vi "rvc Rotation Matrix to RPY.vi"(9 "type of rotations":u16(ring) items=["Extrinsic", "Intrinsic"], 10 "Convension":u16(ring) items=["XYZ", "ZYX"], 11 "rotation matrix":T1) -> (3 "angles":cluster{"roll":dbl, "pitch":dbl, "yaw":dbl})   [LabVIEW 2013]
uses:
  <vilib>/Analysis/Matrix/Datatypes/RealMatrix.ctl
  <vilib>/Analysis/coordinate.llb/Euler Rotation Order.ctl
  <vilib>/robotics/Kinematics/NI_Kinematics.lvlib
  <vilib>/Analysis/NI_AALBase.lvlib
  <vilib>/Analysis/baseanly.llb/Real A x B.vi
  <vilib>/Analysis/NI_AALPro.lvlib
  <vilib>/Analysis/Matrix/NI_Matrix.lvlib
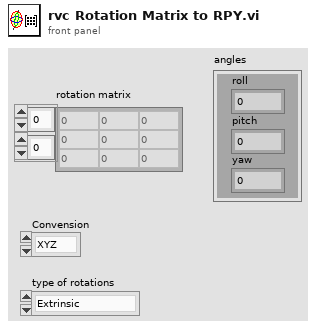
[diagram p1: front panel]
types:
  T1 = typedef "NI_Matrix.lvlib/RealMatrix.ctl" = dbl[][]
  T2 = typedef "NI_AALPro.lvlib/Euler Rotation Order.ctl" = u16
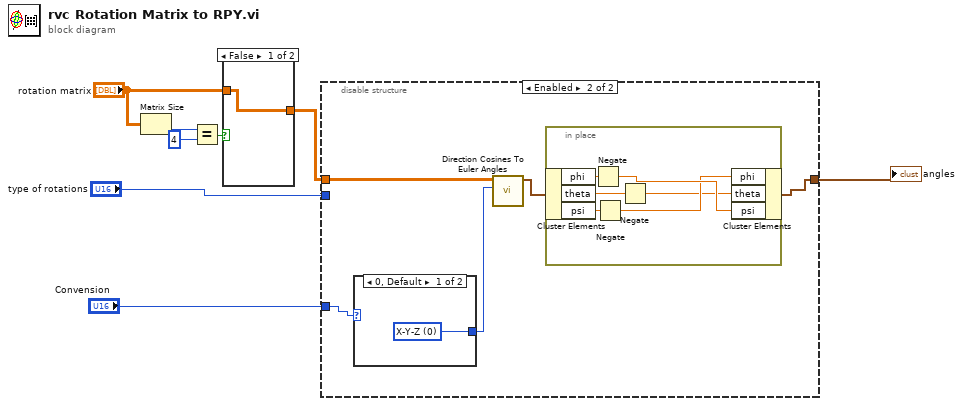
[diagram p0: block diagram]
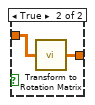
[diagram p2: hidden frame]
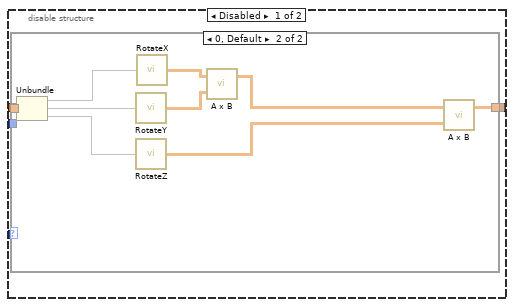
[diagram p3: hidden frame]
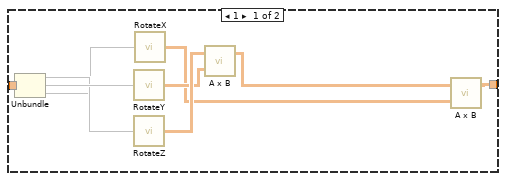
[diagram p4: hidden frame]
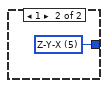
[diagram p5: hidden frame]
diagram:
  n1 = Matrix Size(0:"rotation matrix") -> (2:w5:i32)  [unwired: 1 out]
  n2 = Equal?(x=w5, y=4) -> (x = y?=w3:bool)
  n3 = case shown="False" w3 {
    tunnel: "rotation matrix" -> [w9 w11]
    tunnel: [w9 w10] -> w1
    frame False {
    }
    frame True {
      n4 = call <vilib>:"Transform to Rotation Matrix.vi"("transform"=w11) -> ("rotation matrix"=w10:T1)
    }
  }
  n5 = disable-structure shown="Enabled" {
    disable-tunnel: w1 -> [w14 w36]
    disable-tunnel: [w13 w33] -> w6
    disable-tunnel: "Convension" -> [w12 w37]
    disable-tunnel: "type of rotations" -> [_ _]
    frame Disabled {
      n6 = case shown="0, Default" w12 {
        tunnel: w14 -> [w23 w32]
        tunnel: [w21 w26] -> w13
        frame 1 {
          n7 = Unbundle(w23) -> (w16, w22, w15)
          n8 = call <vilib>:"RotateY.vi"("theta"=w22) -> ("rotation matrix"=w19:T1)
          n9 = call <vilib>:"RotateZ.vi"("theta"=w16) -> ("rotation matrix"=w20:T1)
          n10 = call <vilib>:"RotateX.vi"("theta"=w15) -> ("rotation matrix"=w17:T1)
          n11 = call-poly <vilib>:"A x B.vi"("B"=w19, "A"=w20) -> ("A x B"=w18:T1)  [unwired: 1 out]
          n12 = call-poly <vilib>:"A x B.vi"("B"=w17, "A"=w18) -> ("A x B"=w21:T1)  [unwired: 1 out]
        }
        frame 0, Default {
          n13 = Unbundle(w32) -> (w25, w31, w24)
          n14 = call <vilib>:"RotateY.vi"("theta"=w31) -> ("rotation matrix"=w29:T1)
          n15 = call <vilib>:"RotateZ.vi"("theta"=w24) -> ("rotation matrix"=w28:T1)
          n16 = call <vilib>:"RotateX.vi"("theta"=w25) -> ("rotation matrix"=w30:T1)
          n17 = call-poly <vilib>:"A x B.vi"("B"=w29, "A"=w30) -> ("A x B"=w27:T1)  [unwired: 1 out]
          n18 = call-poly <vilib>:"A x B.vi"("B"=w28, "A"=w27) -> ("A x B"=w26:T1)  [unwired: 1 out]
        }
      }
    }
    frame Enabled {
      n19 = case shown="0, Default" w37 {
        tunnel: [w44 w45] -> w35
        frame 0, Default {
          w44 = T2 0 items=["X-Y-Z", "X-Z-Y", "Y-X-Z", "Y-Z-X", "Z-X-Y", "Z-Y-X", "X-Y-X", "X-Z-X", "Y-X-Y", "Y-Z-Y", "Z-X-Z", "Z-Y-Z"] ("rotation order")
        }
        frame 1 {
          w45 = T2 5 items=["X-Y-Z", "X-Z-Y", "Y-X-Z", "Y-Z-X", "Z-X-Y", "Z-Y-X", "X-Y-X", "X-Z-X", "Y-X-Y", "Y-Z-Y", "Z-X-Z", "Z-Y-Z"] ("rotation order")
        }
      }
      n20 = call <vilib>:"Direction Cosines To Euler Angles.vi"("rotation order"=w35, "Direction Cosines"=w36) -> ("Euler Angles"=w34:cluster{"phi":dbl, "theta":dbl, "psi":dbl})  [unwired: 8 in, 1 out]
      n21 = in-place {
        n22 = in-place-cluster #1(w34) -> ("phi"=w43:dbl, "theta"=w39:dbl, "psi"=w42:dbl)
        n23 = Negate(x=w43) -> (-x=w41:dbl)
        n24 = Negate(x=w42) -> (-x=w40:dbl)
        n25 = Negate(x=w39) -> (-x=w38:dbl)
        n26 = in-place-cluster #1("phi"=w40, "theta"=w38, "psi"=w41) -> (w33:cluster{"phi":dbl, "theta":dbl, "psi":dbl})
      }
    }
  }
  "angles" <- w6
